vi "Test PUBLISH packet.vi"() -> ()   [LabVIEW 2013]
uses:
  Control Packets/PUBLISH/PUBLISH.lvclass
  Control Packets/ControlPacket/QualityOfService -- enum.ctl
  Control Packets/ControlPacket/ControlPacket.lvclass/ControlPacket.ctl
  Control Packets/ControlPacket/ControlPacket.lvclass
panel:
  out "Payload":bool
  out "Quality of Service":bool
  out "Topic Name":bool
  out "Packet ID":u16 format="%04x"
  out "error out":errorcluster
  out "Packet Identifier":bool
  out "Packet type":bool
  out "All packets consumed":bool
  out "Complete Packet":bool
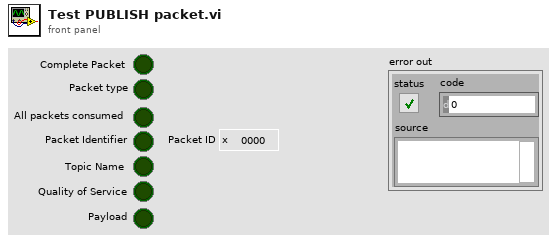
[diagram p1: front panel]
types:
  T1 = typedef "ControlPacket.lvclass/QualityOfService -- enum.ctl" = enum16{"0 (At Most Once)", "1 (At Least Once)", "2 (Exactly Once)"}
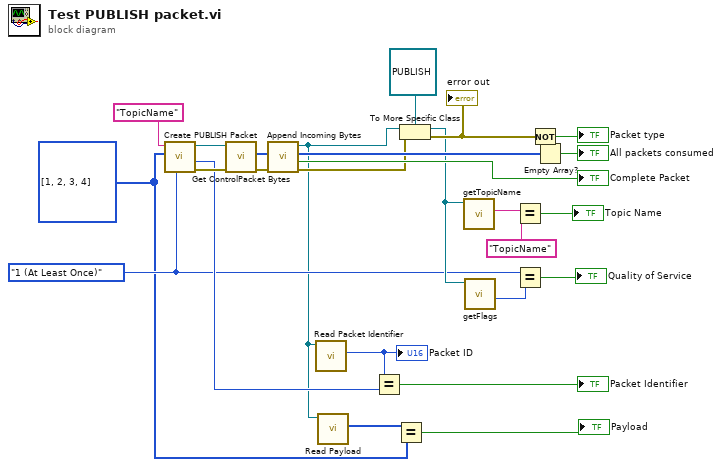
[diagram p0: block diagram]
diagram:
  w2 = u8[] [1, 2, 3, 4] ("Payload")
  w6 = QualityOfService_--_enum."1 (At Least Once)" ("QoS")
  n1 = call "Create PUBLISH Packet.vi"("QoS"=w6, "Payload"=w2, "Topic Name"="TopicName") -> ("error out"=w16:errorcluster, "Packet ID"=w12:u16, "PUBLISH"=w17:refnum<class "PUBLISH.lvclass">)  [unwired: 6 in]
  n2 = call "Get ControlPacket Bytes.vi"("error in (no error)"=w16, "ControlPacket"=w17) -> ("error out"=w20:errorcluster, "Bytes Stream"=w26:u8[])  [unwired: 7 in, 1 out]
  n3 = call "Append Incoming Bytes.vi"("error in (no error)"=w20, "Incoming Packets"=w26) -> ("error out"=w19:errorcluster, "Complete Packet"=→"Complete Packet":bool, "Remaining Packets"=w24:u8[], "ControlPacket"=w4:refnum<class "ControlPacket.lvclass">)  [unwired: 6 in]
  n4 = call "Read Packet Identifier.vi"("ControlPacket in"=w4) -> ("Packet Identifier"=w15:u16)  [unwired: 9 in, 1 out]
  "Packet ID" <- w15
  n5 = call "Read Payload.vi"("ControlPacket in"=w4) -> ("Payload"=w3:u8[])  [unwired: 9 in, 1 out]
  n6 = Equal?(x=w15, y=w12) -> (x = y?=→"Packet Identifier":bool)
  n7 = Equal?(x=w3, y=w2) -> (x = y?=→"Payload":bool)
  n8 = To More Specific Class(target class=refnum<class "PUBLISH.lvclass"> refnum ("PUBLISH.lvclass"), reference=w4, error in=w19) -> (specific class reference=w8:refnum<class "PUBLISH.lvclass">, error out=w22:errorcluster)
  "error out" <- w22
  n9 = call "getTopicName.vi"("PUBLISH in"=w8) -> ("Topic"=w11:string)  [unwired: 8 in, 2 out]
  n10 = call-dynamic "getFlags.vi"("PUBLISH in"=w8) -> ("QoS"=w7:T1)  [unwired: 7 in, 3 out]
  n11 = Equal?(x=w11, y="TopicName" ("Topic Name")) -> (x = y?=→"Topic Name":bool)
  n12 = Equal?(x=w6, y=w7) -> (x = y?=→"Quality of Service":bool)
  n13 = Not(x=w22) -> (.not. x?=→"Packet type":bool)
  n14 = Empty Array?(array=w24) -> (empty?=→"All packets consumed":bool)
